vi "InitBeamShaper.vi"(0 "HasoSlopes in":refnum<class "HasoSlopes.lvclass">, 1 "CorrectionDataManager (const)":refnum<class "CorrectionDataManager.lvclass">, 2 "Pupil (const)":refnum<class "Pupil.lvclass">, 3 "WavefrontCorrector in":refnum<class "WavefrontCorrector.lvclass">, 4 "ComputePhaseSet":refnum<class "ComputePhaseSet.lvclass">, 5 "error in (no error)":errorcluster, 6 "WavefrontCorrectorFilePath":path, 7 "ModalCoef (const)":refnum<class "ModalCoef.lvclass">, 8 "HasoConfigFilePath":path, 9 "InteractionMatrixFilePath":path) -> (10 "CorrectionDataManager out":refnum<class "CorrectionDataManager.lvclass">, 12 "Pupil.lvclass":refnum<class "Pupil.lvclass">, 13 "radius":sgl, 14 "HasoSlopes out":refnum<class "HasoSlopes.lvclass">, 15 "WavefrontCorrector out":refnum<class "WavefrontCorrector.lvclass">, 16 "ComputePhaseSet (new)":refnum<class "ComputePhaseSet.lvclass">, 17 "ModalCoef (new)":refnum<class "ModalCoef.lvclass">, 18 "center":T1, 19 "error out":errorcluster)   [LabVIEW 2020, in "ILAO_BeamShaper.lvclass"]
uses:
  ILAO_BeamShaper.lvclass
  HASO4_3/WaveKit/Controls/Point2Df.ctl
  HASO4_3/WaveKit/Classes/ModalCoef/ModalCoef.lvclass
  HASO4_3/WaveKit/Classes/WavefrontCorrector/WavefrontCorrector.lvclass
  HASO4_3/WaveKit/Classes/ComputePhaseSet/ComputePhaseSet.lvclass
  HASO4_3/WaveKit/Classes/Pupil/Pupil.lvclass
  HASO4_3/WaveKit/Classes/CorrectionDataManager/CorrectionDataManager.lvclass
  HASO4_3/WaveKit/Classes/HasoSlopes/HasoSlopes.lvclass
  HASO4_3/WaveKit/Controls/CircularPupilDetectionParams.ctl
  HASO4_3/WaveKit/Controls/PupilDetectionOption.ctl
  HASO4_3/WaveKit/Controls/CircularAutoDetectionOptions.ctl
  HASO4_3/WaveKit/Controls/PupilDetectionMode.ctl
  HASO4_3/WaveKit/Controls/WavefrontModalReconstructionType.ctl
  HASO4_3/WaveKit/Controls/WavefrontReconstructionMode.ctl
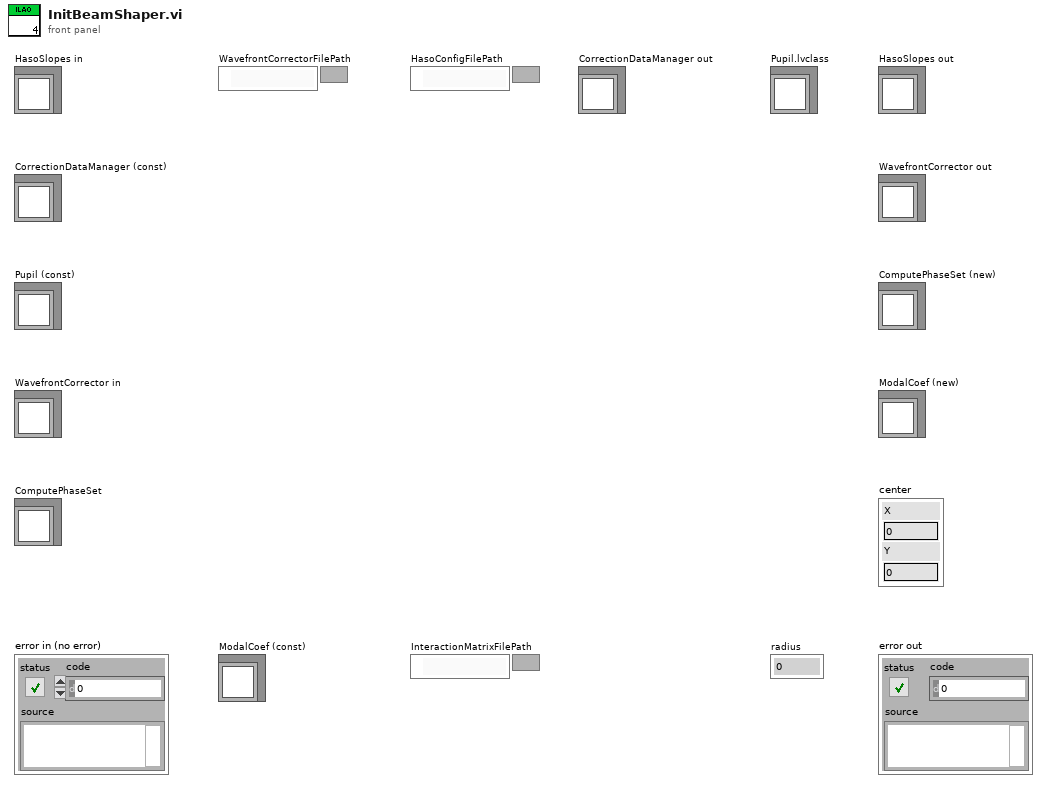
[diagram p1: front panel]
types:
  T1 = typedef "Point2Df.ctl" = cluster{"X":sgl, "Y":sgl}
  T2 = typedef "WavefrontReconstructionMode.ctl" = enum16{"None", "Modal_Legendre", "Modal_Zernike", "Zonal", "Modal_Zonal_Zernike", "Modal_Zonal_Legendre"}
  T3 = typedef "WavefrontModalReconstructionType.ctl" = enum16{"Legendre", "Zernike"}
  T4 = typedef "CircularPupilDetectionParams.ctl" = cluster{"PupilDetectionOption":T5, "AutoDetectionOption":T6, "PupilDetectionMode":T7, "CentralOccultationDetection":bool}
  T5 = typedef "PupilDetectionOption.ctl" = enum16{"Manual", "Automatic"}
  T6 = typedef "CircularAutoDetectionOptions.ctl" = enum16{"manual_radius_auto_center", "manual_center_auto_radius", "auto_radius_auto_center"}
  T7 = typedef "PupilDetectionMode.ctl" = enum16{"inscribed", "circumscribed"}
  T8 = typedef "CasaoManagerGeneralSpecifications.ctl" = cluster{"Wavefront corrector name":string, "Wavefront corrector serial number":string, "Nb actuators":i32, "HASO serial number":string, "Dimension_um":T9}
  T9 = typedef "General dimensions definition.ctl" = cluster{"Size":T10, "Step":T1}
  T10 = typedef "Point2D.ctl" = cluster{"X":u32, "Y":u32}
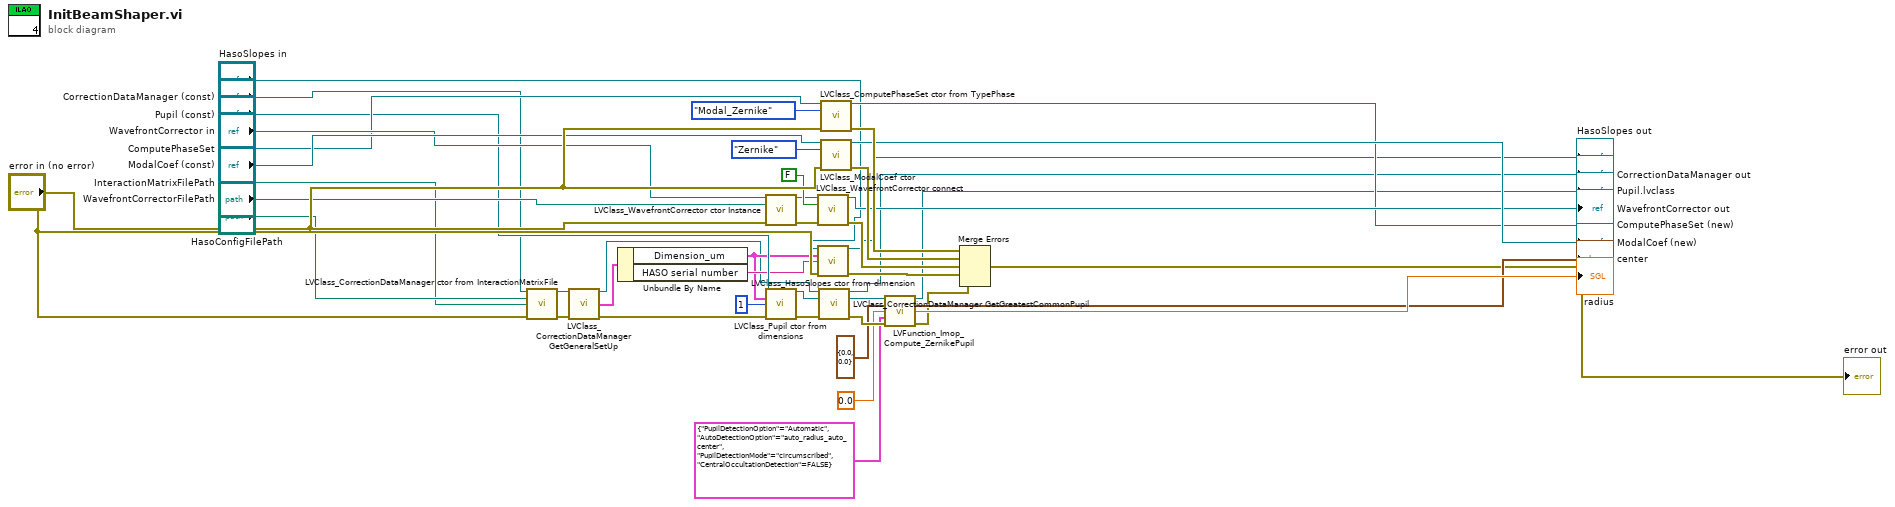
[diagram p0: block diagram]
diagram:
  n1 = call "LVClass_CorrectionDataManager ctor from InteractionMatrixFile.vi"("CorrectionDataManager (const)"="CorrectionDataManager (const)", "Haso config file path"="HasoConfigFilePath", "Interaction matrix path"="InteractionMatrixFilePath", "error in (no error)"="error in (no error)") -> ("CorrectionDataManager (new)"=w1:refnum<class "CorrectionDataManager.lvclass">, "error out"=w2:errorcluster)  [unwired: 10 in]
  n2 = call "LVClass_CorrectionDataManager GetGeneralSetUp.vi"("CorrectionDataManager in"=w1, "error in (no error)"=w2) -> ("CorrectionDataManager out"=w4:refnum<class "CorrectionDataManager.lvclass">, "general"=w3:T8, "error out"=w33:errorcluster)  [unwired: 11 in]
  n3 = Unbundle By Name(w3) -> ("Dimension_um"=w13:T9, "HASO serial number"=w14:string)
  n4 = call "LVClass_WavefrontCorrector ctor Instance.vi"("WavefrontCorrector (const)"="WavefrontCorrector in", "PathToWavefrontCorrectorSetupFile"="WavefrontCorrectorFilePath", "error in (no error)"="error in (no error)") -> ("WavefrontCorrector (new)"=w16:refnum<class "WavefrontCorrector.lvclass">, "error out"=w15:errorcluster)  [unwired: 11 in]
  n5 = call "LVClass_Pupil ctor from dimensions.vi"("Pupil (const)"="Pupil (const)", "Dimensions_um"=w13, "value"=u8 1, "error in (no error)"=w33) -> ("Pupil (new)"=w6:refnum<class "Pupil.lvclass">, "error out"=w34:errorcluster)  [unwired: 10 in]
  n6 = call "LVClass_WavefrontCorrector connect.vi"("WavefrontCorrector in"=w16, "set_init_state_from_config_file"=FALSE, "error in (no error)"=w15) -> ("WavefrontCorrector out"=→"WavefrontCorrector out":refnum<class "WavefrontCorrector.lvclass">, "error out"=w39:errorcluster)  [unwired: 11 in]
  n7 = call "LVClass_HasoSlopes ctor from dimension.vi"("HasoSlopes (const)"="HasoSlopes in", "Dimensions_um"=w13, "serial"=w14, "error in (no error)"="error in (no error)") -> ("HasoSlopes (new)"=→"HasoSlopes out":refnum<class "HasoSlopes.lvclass">, "error out"=w36:errorcluster)  [unwired: 10 in]
  n8 = call "LVClass_CorrectionDataManager GetGreatestCommonPupil.vi"("CorrectionDataManager in"=w4, "Pupil in"=w6, "error in (no error)"=w34) -> ("CorrectionDataManager out"=→"CorrectionDataManager out":refnum<class "CorrectionDataManager.lvclass">, "Pupil out"=w10:refnum<class "Pupil.lvclass">, "error out"=w41:errorcluster)  [unwired: 10 in]
  n9 = call "LVClass_ComputePhaseSet ctor from TypePhase.vi"("ComputePhaseSet (const)"="ComputePhaseSet", "TypePhase"=WavefrontReconstructionMode."Modal_Zernike", "error in (no error)"="error in (no error)") -> ("ComputePhaseSet (new)"=→"ComputePhaseSet (new)":refnum<class "ComputePhaseSet.lvclass">, "error out"=w37:errorcluster)  [unwired: 11 in]
  n10 = call "LVClass_ModalCoef ctor.vi"("ModalCoef (const)"="ModalCoef (const)", "TypePhase"=WavefrontModalReconstructionType."Zernike", "error in (no error)"="error in (no error)") -> ("ModalCoef (new)"=→"ModalCoef (new)":refnum<class "ModalCoef.lvclass">, "error out"=w38:errorcluster)  [unwired: 11 in]
  n11 = call "LVFunction_Imop_Compute_ZernikePupil.vi"("Pupil.lvclass"=w10, "center in"=T1 {"X"=0.0, "Y"=0.0}, "radius in"=sgl 0.0, "CircularPupilDetectionParams"=T4 {"PupilDetectionOption"=enum."Automatic", "AutoDetectionOption"=enum."auto_radius_auto_center", "PupilDetectionMode"=enum."circumscribed", "CentralOccultationDetection"=FALSE}, "error in"=w41) -> ("Pupil.lvclass"=→"Pupil.lvclass":refnum<class "Pupil.lvclass">, "center"=→"center":T1, "radius"=→"radius":sgl, "error out"=w42:errorcluster)  [unwired: 7 in]
  n12 = Merge Errors(w37, w38, w39, w36, w42) -> (→"error out":errorcluster)
